vi "GUI Login Window.vi"(10 "Password in":string caption="Senha", 11 "FOFB-Controller IP Address in":string caption="Endereço IP do controlador do FOFB") -> (1 "Cancelled?":bool, 2 "Password out":string="boo500mev", 3 "FOFB-Controller IP Address out":string="10.0.5.31")   [LabVIEW 2011, in "User Interface Window VIs.lvlib"]
uses:
  User Interface Window VIs.lvlib
panel:
  in  "Cancel":bool
  in  "OK Button":bool
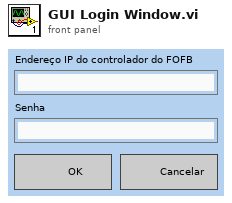
[diagram p1: front panel]
types:
  T1 = typedef "eventvkey.ctl" = enum16{"ASCII", "Enter", "Return", "Shift", "Ctrl", "Alt", "Cmd", "Opt", "Caps", "NumLock", "Clear", "Break", "Up", "Down", "Left", "Right", "Insert", "Delete", "Home", "End", "PageUp", "PageDown", "Escape", "Help", "Pause", "ScrollLock", "F1", "F2", "F3", "F4", "F5", "F6", "F7", "F8", "F9", "F10", "F11", "F12", "F13", "F14", "F15", "F16", "F17", "F18", "F19", "F20", "F21", "F22", "F23", "F24", "Play", "VolumeUp", "VolumeDown", "Mute", "Two Byte Char"}
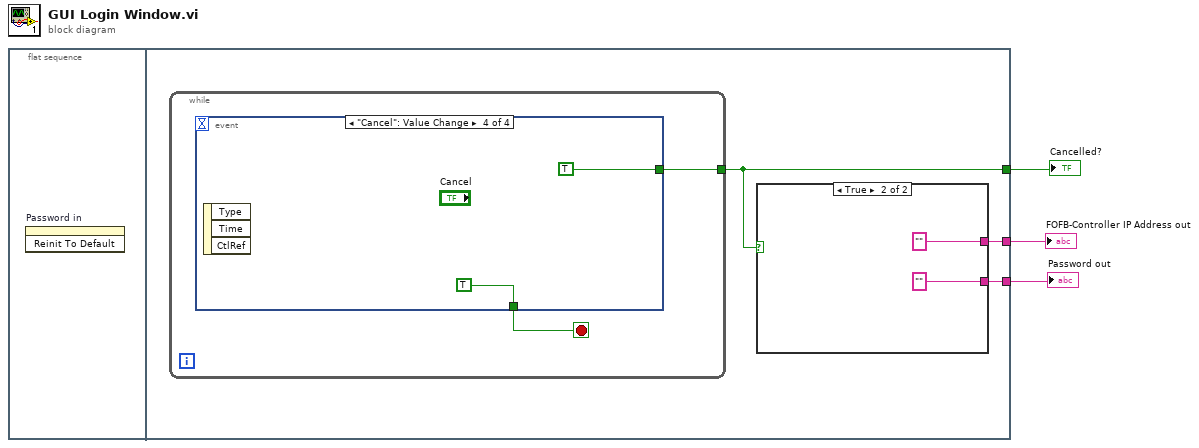
[diagram p0: block diagram]
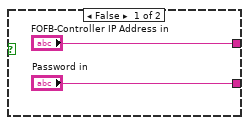
[diagram p2: hidden frame]
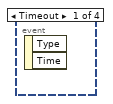
[diagram p3: hidden frame]
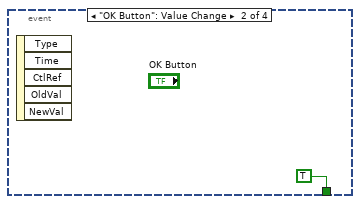
[diagram p4: hidden frame]
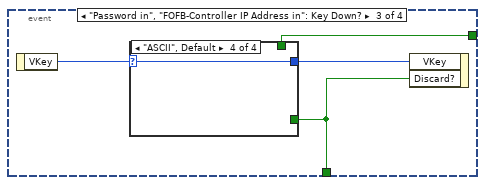
[diagram p5: hidden frame]
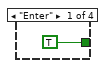
[diagram p6: hidden frame]
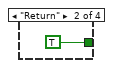
[diagram p7: hidden frame]
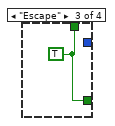
[diagram p8: hidden frame]
diagram:
  n1 = flat-sequence {
    tunnel: [w6] -> w3
    tunnel: [w5] -> w2
    tunnel: [w4] -> w1
    frame #0 {
      n2 = invoke on="Password in" class="Str" method="Reinit To Default"() -> ()  [unwired: 3 in, 3 out]
    }
    frame #1 {
      n3 = while {
        tunnel: [w12] -> w6
        stop <- w11 stop-if-true
        n4 = event shown="[3] \"Cancel\": Value Change" {
          selector: _ -> [_ _ _ _]
          dyn-events: _ -> [_ _ _ _]
          timeout: _ -> [_ _ _ _]
          tunnel: [_ _ w17 TRUE ("Cancel")] -> w12
          tunnel: [_ TRUE ("Cancel") w14 TRUE ("Cancel")] -> w11
          event Timeout {
            n5 = event-data() -> ()  [unwired: 1 in, 2 out]
          }
          event "OK Button": Value Change {
            n6 = event-data() -> ()  [unwired: 1 in, 5 out]
          }
          event "Password in", "FOFB-Controller IP Address in": Key Down? {
            n7 = event-data() -> ("VKey"=w16:T1)  [unwired: 1 in]
            n8 = case shown="\"ASCII\", Default" w16 {
              selector: w16 -> [_ _ _ w21]
              tunnel: [TRUE ("Discard?") TRUE ("Discard?") w20 _] -> w14
              tunnel: [_ _ w20 _] -> w17
              tunnel: [_ _ _ w21] -> w15
              frame "Enter" {
              }
              frame "Return" {
              }
              frame "Escape" {
                w20 = TRUE ("Discard?")
              }
              frame "ASCII", Default {
              }
            }
            n9 = event-data("VKey"=w15, "Discard?"=w14) -> ()  [unwired: 1 in, 1 out]
          }
          event "Cancel": Value Change {
            n10 = event-data() -> ()  [unwired: 1 in, 3 out]
          }
        }
      }
      n11 = case shown="True" w6 {
        tunnel: ["FOFB-Controller IP Address in" "" ("FOFB-Controller IP Address in")] -> w5
        tunnel: ["Password in" "" ("Password in")] -> w4
        frame False {
        }
        frame True {
        }
      }
    }
  }
  "Password out" <- w1
  "FOFB-Controller IP Address out" <- w2
  "Cancelled?" <- w3
